vi "Write Send Period (ms).vi"(8 "error in (no error)":errorcluster, 10 "Send Period (ms)":i32=1000, 11 "Sender Loop in":refnum<class "Sender Loop.lvclass">) -> (0 "error out":errorcluster, 3 "Sender Loop out":refnum<class "Sender Loop.lvclass">)   [LabVIEW 2021, in "Secure Echo Broadcast With Server Manager.lvlib" / "Sender Loop.lvclass"]
uses:
  Sender Loop.lvclass
  Sender Loop.lvclass/Sender Loop.ctl
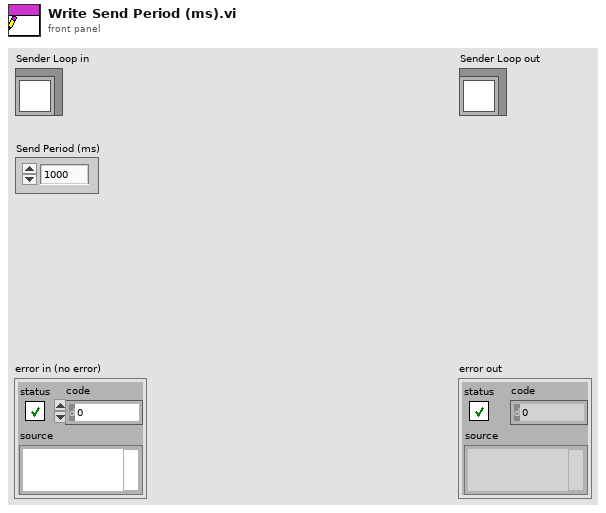
[diagram p1: front panel]
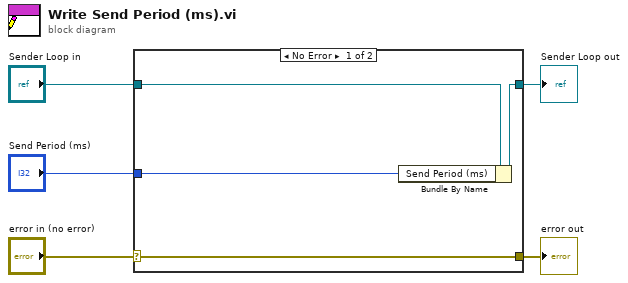
[diagram p0: block diagram]
diagram:
  n1 = case shown="No Error" "error in (no error)" {
    selector: "error in (no error)" -> [w9 w10]
    tunnel: [w9 w10] -> w4
    tunnel: [w7 w11] -> w2
    tunnel: "Sender Loop in" -> [w8 w11]
    tunnel: "Send Period (ms)" -> [w6 _]
    frame No Error {
      n2 = Bundle By Name(cluster=w8, "Send Period (ms)"=w6) -> (w7:refnum<class "Sender Loop.lvclass">)
    }
    frame Error {
    }
  }
  "error out" <- w4
  "Sender Loop out" <- w2
